vi "R2R-Controller-PCTesting.vi"(4 "Custom Controller Inputs":T1, 6 "Gain Configuration":T2={"PID Gains"={"proportional gain (Kc)"=1.0, "integral gain (Kc*Ts/Ti)"=0.0, "derivative gain (Kc*Td/Ts)"=0.0}, "Output Range"={"output high"=10.0, "output low"=-10.0}}, 7 "Reset Integrator":bool, 8 "X (Raw Analog V)":fxp<+,18,3>, 9 "F (Raw Analog V)":fxp<+,18,3>, 10 "X* (mm)":fxp<+/-,16,7>, 11 "F* (N)":fxp<+/-,16,7>) -> (0 "X(mm)":fxp<+,30,7>, 1 "Measured Force (N)":fxp<+,39,10>, 2 "V*(V)":fxp<+/-,53,13> format="%.6f", 3 "PWM Duty Cycle":i16, 5 "Duty Cycle Output":i16)   [LabVIEW 2013]
uses:
  controls/Control Configuration.ctl
  controls/Custom Controller Inputs.ctl
  <vilib>/rvi/Analysis/measure/butterworth/XNode/niFpgaButterworthFilter.xnode
  <vilib>/addons/control/pid/fpga.llb/XNode/niFpgaPID.xnode
panel:
  in  "F deadband thresh (N)":fxp<+/-,16,5>=1.0
  out "Y*'":fxp<+/-,36,31>
  out "Y*":fxp<+/-,64,27>
  in  "K_PosSense (mm/Volt)":fxp<+,12,4>=10.0
  out "DeltaX*":fxp<+/-,32,11>
  out "F_Error (N)":fxp<+/-,40,11>
  in  "K_PWM (Counts/Volt)":fxp<+,16,7>=83.33203125
  in  "Ra (Armature Resistance) (Ohms)":fxp<+/-,7,7>=60.0
  out "I* Current Command (A)":fxp<+,18,3>
  in  "Force Sensor Gain (N/V)":fxp<+,20,6>=53.02703857421875
  in  "L12 Gain (mA/N)":fxp<+,16,2>=2.29180908203125
  in  "L12 Offset (mA)":fxp<+,18,4>=12.9949951171875
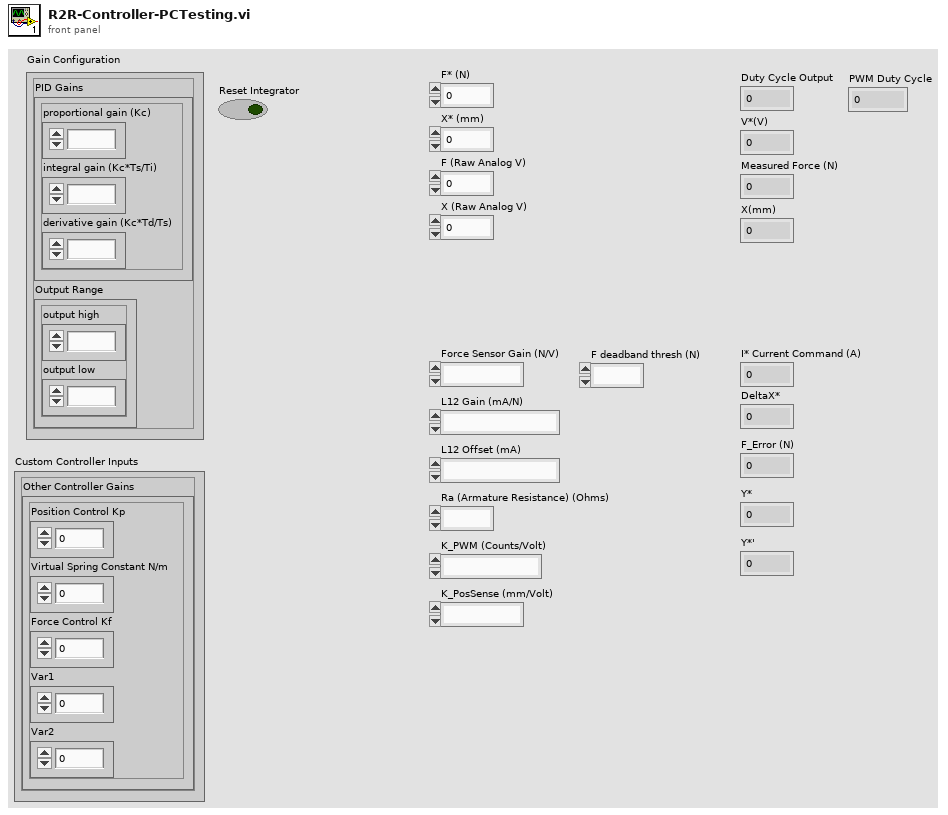
[diagram p1: front panel]
types:
  T1 = typedef "Custom Controller Inputs.ctl" = cluster{"Other Controller Gains":cluster{"Position Control Kp":fxp<+/-,16,8>, "Virtual Spring Constant N/m":fxp<+,16,12>, "Force Control Kf":fxp<+/-,16,8>, "Var1":fxp<+/-,16,5>, "Var2":fxp<+/-,16,5>}}
  T2 = typedef "Control Configuration.ctl" = cluster{"PID Gains":cluster{"proportional gain (Kc)":fxp<+/-,16,8>, "integral gain (Kc*Ts/Ti)":fxp<+/-,16,8>, "derivative gain (Kc*Td/Ts)":fxp<+/-,16,8>}, "Output Range":cluster{"output high":fxp<+/-,16,7>, "output low":fxp<+/-,16,7>}}
  T3 = cluster{"Position Control Kp":fxp<+/-,16,8>, "Virtual Spring Constant N/m":fxp<+,16,12>, "Force Control Kf":fxp<+/-,16,8>, "Var1":fxp<+/-,16,5>, "Var2":fxp<+/-,16,5>}
  T4 = cluster{"proportional gain (Kc)":fxp<+/-,16,8>, "integral gain (Kc*Ts/Ti)":fxp<+/-,16,8>, "derivative gain (Kc*Td/Ts)":fxp<+/-,16,8>}
  T5 = cluster{"output high":fxp<+/-,16,7>, "output low":fxp<+/-,16,7>}
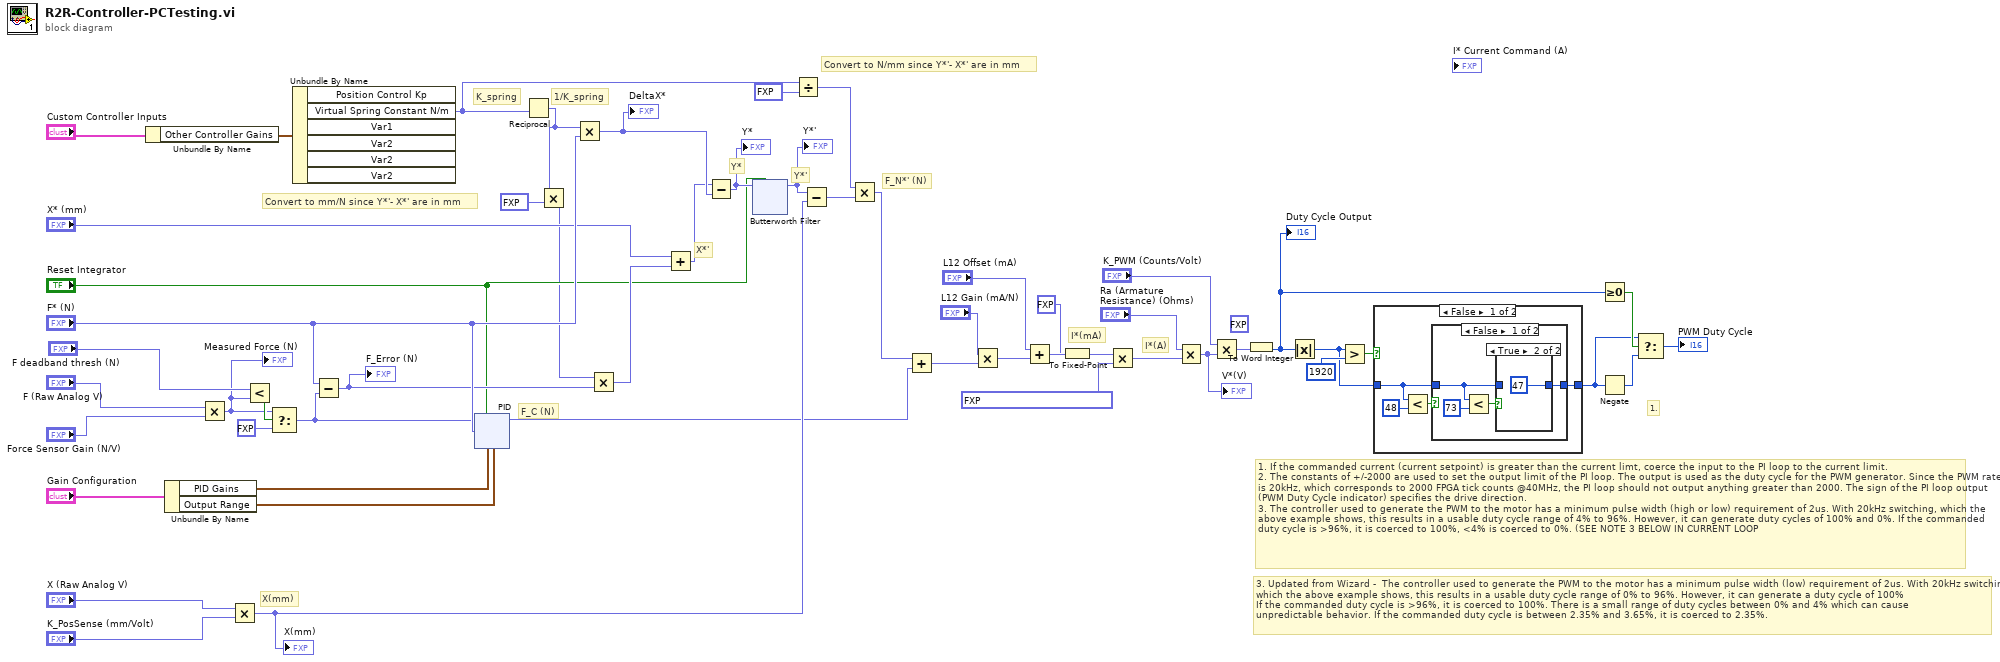
[diagram p0: block diagram]
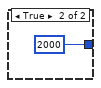
[diagram p4: hidden frame]
diagram:
  (unwired) fxp<+/-,16,16> 0.0 ("fixed-point type")
  # "Convert to mm/N since Y*'- X*' are in mm"
  # "Convert to N/mm since Y*'- X*' are in mm"
  # "1. If the commanded current (current setpoint) is greater than the current limt, coerce the input to the PI loop to the current limit.\n2. The constants of +/-2000 are used to set the output limit of the PI loop. The output is used as the duty cycle for the PWM generator. Since the PWM rate is 20kHz, which corresponds to 2000 FPGA tick counts @40MHz, the PI loop should not output anything greater than 2000. The sign of the PI loop output (PWM Duty Cycle indicator) specifies the drive direction.\n3. The controller used to generate the PWM to the motor has a minimum pulse width (high or low) requirement of 2us. With 20kHz switching, which the above example shows, this results in a usable duty cycle range of 4% to 96%. However, it can generate duty cycles of 100% and 0%. If the commanded duty cycle is >96%, it is coerced to 100%, <4% is coerced to 0%. (SEE NOTE 3 BELOW IN CURRENT LOOP"
  # "3. Updated from Wizard -  The controller used to generate the PWM to the motor has a minimum pulse width (low) requirement of 2us. With 20kHz switching, which the above example shows, this results in a usable duty cycle range of 0% to 96%. However, it can generate a duty cycle of 100%\nIf the commanded duty cycle is >96%, it is coerced to 100%. There is a small range of duty cycles between 0% and 4% which can cause\nunpredictable behavior. If the commanded duty cycle is between 2.35% and 3.65%, it is coerced to 2.35%."
  # "1."
  # "Y*'"
  # "I*(A)"
  # "I*(mA)"
  # "F_C (N)"
  # "F_N*' (N)"
  # "X(mm)"
  # "Y*"
  # "X*'"
  # "K_spring"
  # "1/K_spring"
  n1 = Unbundle By Name("Custom Controller Inputs") -> ("Other Controller Gains"=w48:T3)
  n2 = Unbundle By Name("Gain Configuration") -> ("PID Gains"=w52:T4, "Output Range"=w51:T5)
  n3 = Multiply(x="F (Raw Analog V)", y="Force Sensor Gain (N/V)") -> (x*y=w5:fxp<+,38,9>)
  "Measured Force (N)" <- w5
  n4 = Multiply(x="X (Raw Analog V)", y="K_PosSense (mm/Volt)") -> (x*y=w38:fxp<+,30,7>)
  "X(mm)" <- w38
  n5 = Less?(x="F deadband thresh (N)", y=w5) -> (x < y?=w6:bool)
  n6 = Select(t=w5, s=w6, f=fxp<+,38,9> 0.0) -> (s? t:f=w3:fxp<+,38,9>)
  n7 = Unbundle By Name(w48) -> ("Virtual Spring Constant N/m"=w36:fxp<+,16,12>)  [unwired: 5 out]
  n8 = Subtract(x="F* (N)", y=w3) -> (x-y=w46:fxp<+/-,40,11>)
  "F_Error (N)" <- w46
  n9 = xnode "PID"("process variable"=w3, "reset?"="Reset Integrator", "setpoint"="F* (N)", "PID gains"=w52, "output range"=w51) -> ("output"=w34:fxp<+/-,16,10>)
  n10 = Reciprocal(x=w36) -> (1/x=w45:fxp<+,17,5>)
  n11 = Multiply(x=w45, y=fxp<+,17,10> 1000.0) -> (x*y=w12:fxp<+,33,14>)
  n12 = Multiply(x=w45, y="F* (N)") -> (x*y=w42:fxp<+/-,32,11>)
  "DeltaX*" <- w42
  n13 = Multiply(x=w12, y=w46) -> (x*y=w43:fxp<+/-,64,25>)
  n14 = Add(x="X* (mm)", y=w43) -> (x+y=w41:fxp<+/-,64,26>)
  n15 = Subtract(x=w41, y=w42) -> (x-y=w24:fxp<+/-,64,27>)
  "Y*" <- w24
  n16 = xnode "Butterworth Filter"("input data"=w24, "reset"="Reset Integrator") -> ("output data"=w23:fxp<+/-,36,31>)  [unwired: 1 in]
  "Y*'" <- w23
  n17 = Divide(x=w36, y=fxp<+,16,12> 1000.0) -> (x/y=w14:fxp<+,32,16>)
  n18 = Subtract(x=w23, y=w38) -> (x-y=w37:fxp<+/-,55,32>)
  n19 = Multiply(x=w14, y=w37) -> (x*y=w35:fxp<+/-,64,47>)
  n20 = Add(x=w35, y=w34) -> (x+y=w32:fxp<+/-,64,48>)
  n21 = Multiply(x="L12 Gain (mA/N)", y=w32) -> (x*y=w31:fxp<+/-,64,50>)
  n22 = Add(x="L12 Offset (mA)", y=w31) -> (x+y=w10:fxp<+/-,64,51>)
  n23 = To Fixed-Point(fixed-point type=fxp<+/-,32,16> 0.0, number=w10) -> (fixed-point=w8:fxp<+/-,32,16>)
  n24 = Multiply(x=w8, y=fxp<+/-,16,-8> 0.0009999871253967285) -> (x*y=w28:fxp<+/-,48,8>)
  n25 = Multiply(x="Ra (Armature Resistance) (Ohms)", y=w28) -> (x*y=w26:fxp<+/-,53,13>)
  "V*(V)" <- w26
  n26 = Multiply(x="K_PWM (Counts/Volt)", y=w26) -> (x*y=w2:fxp<+/-,64,20>)
  n27 = To Word Integer(number=w2) -> (16bit integer=w1:i16)
  "Duty Cycle Output" <- w1
  n28 = Absolute Value(x=w1) -> (abs(x)=w16:i16)
  n29 = Greater?(x=w16, y=i16 1920 ("upper limit")) -> (0:w18:bool)
  n30 = case shown="False" w18 {
    tunnel: [w57 i16 2000 ("upper limit")] -> w17
    tunnel: w16 -> [w55 _]
    frame False {
      n31 = Less?(x=w55, y=i16 48 ("lower limit")) -> (x < y?=w56:bool)
      n32 = case shown="False" w56 {
        tunnel: [w59 w65] -> w57
        tunnel: w55 -> [w60 w65]
        frame False {
          n33 = Less?(x=w60, y=i16 73 ("lower limit")) -> (x < y?=w61:bool)
          n34 = case shown="True" w61 {
            tunnel: w60 -> [w63 _]
            tunnel: [w63 i16 47 ("lower limit")] -> w59
            frame False {
            }
            frame True {
            }
          }
        }
        frame True {
        }
      }
    }
    frame True {
    }
  }
  n35 = Greater Or Equal To 0?(x=w1) -> (x >= 0?=w21:bool)
  n36 = Negate(x=w17) -> (-x=w20:i16)
  n37 = Select(t=w17, s=w21, f=w20) -> (s? t:f=→"PWM Duty Cycle":i16)
